vi "Dispenser Low Level.vi"(8 "error in (no error)":errorcluster, 9 "Bottom Pin":tag, 10 "Top Pin":tag="B/PWM0", 11 "Function":T1) -> (0 "error out":errorcluster)   [LabVIEW 2014]
uses:
  Controls/Dispenser Functions.ctl
  <vilib>/myRIO/Common/Instrument Driver Framework/myRIO v1.0/PWM/vis/myRIO v1.1 Open PWM.vi
  <vilib>/myRIO/Common/Instrument Driver Framework/Utilities/vis/Validate Channels.vi
  <vilib>/myRIO/Common/Instrument Driver Framework/myRIO v1.0/PWM/vis/myRIO v1.0 Reserve PWM.vi
  <vilib>/myRIO/Common/Instrument Driver Framework/myRIO v1.0/PWM/vis/myRIO v1.0 Build MUX Configuration PWM.vi
  <vilib>/myRIO/Common/Instrument Driver Framework/myRIO v1.0/Resource Manager/vis/myRIO v1.0 Reserve Channel List.vi
  <vilib>/myRIO/Common/Instrument Driver Framework/myRIO v1.0/Resource Manager/vis/myRIO v1.0 Create Configuration List.vi
  <vilib>/myRIO/Common/Instrument Driver Framework/myRIO v1.0/Resource Manager/vis/myRIO v1.0 Reserve Channel.vi
  <vilib>/myRIO/Common/Instrument Driver Framework/myRIO v1.0/Resource Manager/vis/myRIO v1.0 Unreserve Channel.vi
  <vilib>/myRIO/Common/Instrument Driver Framework/myRIO v1.0/Resource Manager/vis/myRIO v1.0 Build Mutex Name.vi
  <vilib>/Utility/VariantDataType/GetNumericInfo.vi
  <vilib>/Utility/error.llb/Error Cluster From Error Code.vi
  <vilib>/myRIO/Common/Instrument Driver Framework/myRIO v1.0/myRIO v1.1 Open.vi
  <vilib>/myRIO/Common/Instrument Driver Framework/Utilities/vis/IO Manager.vi
  <vilib>/myRIO/Common/Instrument Driver Framework/Utilities/vis/Configuration Manager.vi
  <vilib>/myRIO/Common/Instrument Driver Framework/myRIO v1.0/Resource Manager/vis/myRIO v1.0 Configure IO.vi
  <vilib>/myRIO/Common/Instrument Driver Framework/myRIO v1.0/myRIO v1.0 Close.vi
  <vilib>/myRIO/Common/Instrument Driver Framework/myRIO v1.0/PWM/vis/myRIO v1.0 Write PWM.vi
  <vilib>/myRIO/Instrument Drivers/Onboard IO/PWM/PWM.lvlib
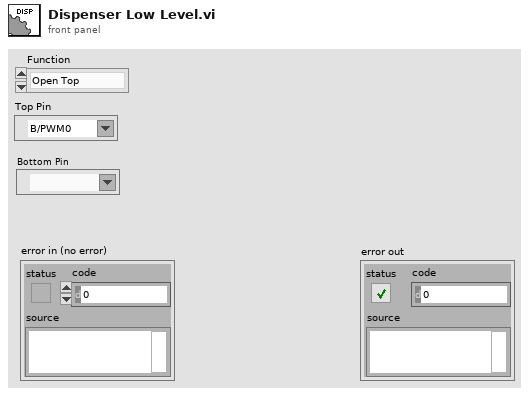
[diagram p1: front panel]
types:
  T1 = typedef "Dispenser Functions.ctl" = enum16{"Open Top", "Close Top", "Close Bottom", "Open Bottom"}
  T2 = typedef "PWM.lvlib/PWM Reference.ctl" = cluster{"myRIO Reference":T3, "PWM Channels Enum":T7, "PWM Configuration":T8}
  T3 = typedef "myRIO Generic Hardware Reference.ctl" = cluster{"myRIO Model":T4, "myRIO Hardware Reference":T5}
  T4 = typedef "Hardware Version Enum.ctl" = enum16{"Unknown", "myRIO-1900", "myRIO-1950"}
  T5 = typedef "myRIO v1.0 Reference.ctl" = cluster{"Generic FPGA Reference":T6, "Allow multiple opens":bool}
  T6 = typedef "Generic FPGA Reference.ctl" = refnum<k20>
  T7 = typedef "PWM Channels Enum.ctl" = enum16{"Not Connected", "C/PWM0", "C/PWM1", "A/PWM0", "A/PWM1", "A/PWM2", "B/PWM0", "B/PWM1", "B/PWM2"}
  T8 = typedef "PWM.lvlib/PWM Configuration.ctl" = cluster{"Frequency":dbl, "Duty Cycle":dbl}
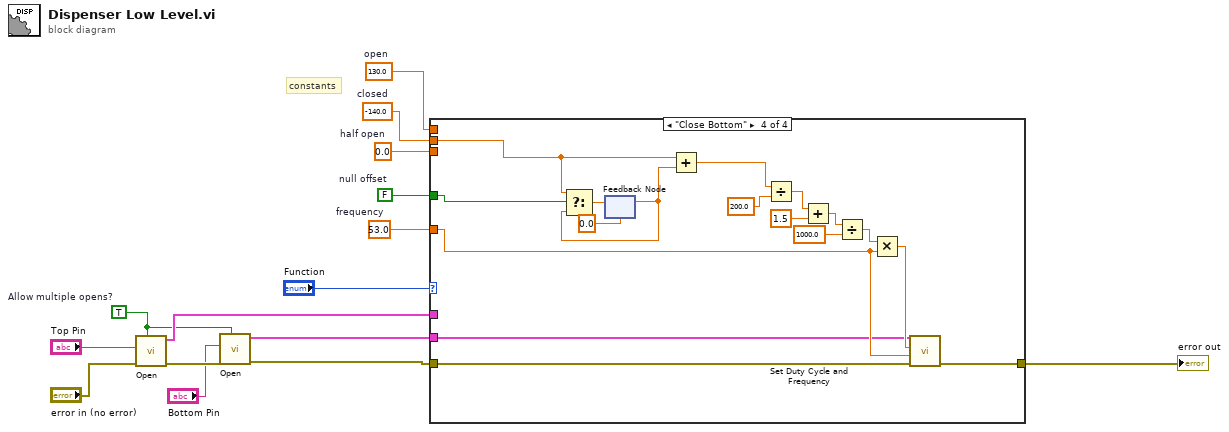
[diagram p0: block diagram]
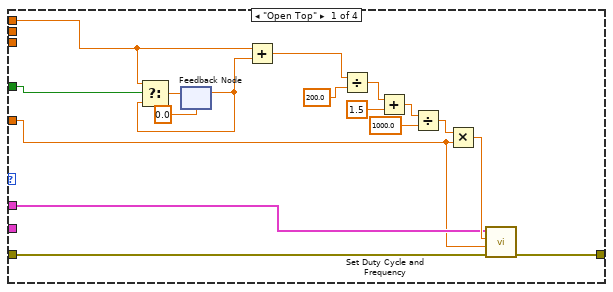
[diagram p2: hidden frame]
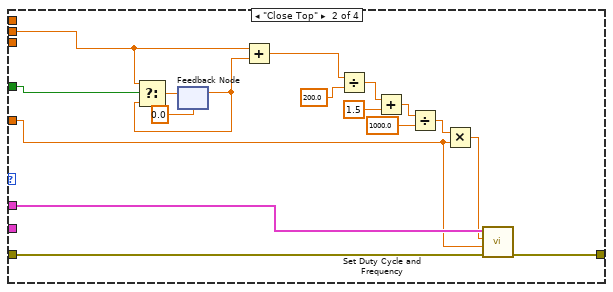
[diagram p3: hidden frame]
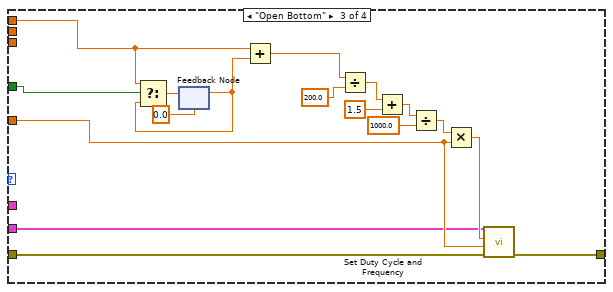
[diagram p4: hidden frame]
diagram:
  w2 = TRUE  # Allow multiple opens?
  w5 = FALSE  # null offset
  w6 = 53.0  # frequency
  w7 = 0.0  # half open
  w9 = -140.0  # closed
  w8 = 130.0  # open
  # "constants"
  n1 = call <vilib>:"Open.vi"("Allow multiple opens?"=w2, "error in (no error)"="error in (no error)", "Channel Name"="Top Pin") -> ("error out"=w12:errorcluster, "PWM Ref Out"=w3:T2)  [unwired: 7 in]
  n2 = call <vilib>:"Open.vi"("Allow multiple opens?"=w2, "error in (no error)"=w12, "Channel Name"="Bottom Pin") -> ("error out"=w11:errorcluster, "PWM Ref Out"=w4:T2)  [unwired: 7 in]
  n3 = case shown="\"Close Bottom\"" "Function" {
    tunnel: w3 -> [w19 w44 _ _]
    tunnel: w11 -> [w20 w43 w54 w72]
    tunnel: [w21 w36 w55 w71] -> w1
    tunnel: w4 -> [_ _ w50 w67]
    tunnel: w9 -> [_ w35 _ w68]
    tunnel: w8 -> [w18 _ w53 _]
    tunnel: w7 -> [_ _ _ _]
    tunnel: w6 -> [w16 w34 w51 w70]
    tunnel: w5 -> [w17 w33 w52 w69]
    frame "Open Top" {
      n4 = feedback #1(0.0 ("position [%FS]")) -> (w29:dbl)
      n5 = Select(t=w18, s=w17, f=w29) -> (s? t:f=w27:dbl)
      n6 = feedback-in #1(w27) -> ()
      n7 = Add(x=w18, y=w29) -> (x+y=w28:dbl)
      n8 = Divide(x=w28, y=200.0) -> (x/y=w23:dbl)
      n9 = Add(x=w23, y=1.5) -> (x+y=w25:dbl)
      n10 = Divide(x=w25, y=1000.0) -> (x/y=w30:dbl)
      n11 = Multiply(x=w30, y=w16) -> (x*y=w31:dbl)
      n12 = call <vilib>:"Set Duty Cycle and Frequency.vi"("error in (no error)"=w20, "Frequency [Hz]"=w16, "Duty Cycle"=w31, "PWM Ref In"=w19) -> ("error out"=w21:errorcluster)  [unwired: 5 in, 1 out]
    }
    frame "Close Top" {
      n13 = feedback #2(0.0 ("position [%FS]")) -> (w40:dbl)
      n14 = Select(t=w35, s=w33, f=w40) -> (s? t:f=w42:dbl)
      n15 = feedback-in #2(w42) -> ()
      n16 = Add(x=w35, y=w40) -> (x+y=w41:dbl)
      n17 = Divide(x=w41, y=200.0) -> (x/y=w48:dbl)
      n18 = Add(x=w48, y=1.5) -> (x+y=w46:dbl)
      n19 = Divide(x=w46, y=1000.0) -> (x/y=w39:dbl)
      n20 = Multiply(x=w39, y=w34) -> (x*y=w38:dbl)
      n21 = call <vilib>:"Set Duty Cycle and Frequency.vi"("error in (no error)"=w43, "Frequency [Hz]"=w34, "Duty Cycle"=w38, "PWM Ref In"=w44) -> ("error out"=w36:errorcluster)  [unwired: 5 in, 1 out]
    }
    frame "Open Bottom" {
      n22 = feedback #3(0.0 ("position [%FS]")) -> (w63:dbl)
      n23 = Select(t=w53, s=w52, f=w63) -> (s? t:f=w61:dbl)
      n24 = feedback-in #3(w61) -> ()
      n25 = Add(x=w53, y=w63) -> (x+y=w62:dbl)
      n26 = Divide(x=w62, y=200.0) -> (x/y=w57:dbl)
      n27 = Add(x=w57, y=1.5) -> (x+y=w59:dbl)
      n28 = Divide(x=w59, y=1000.0) -> (x/y=w64:dbl)
      n29 = Multiply(x=w64, y=w51) -> (x*y=w65:dbl)
      n30 = call <vilib>:"Set Duty Cycle and Frequency.vi"("error in (no error)"=w54, "Frequency [Hz]"=w51, "Duty Cycle"=w65, "PWM Ref In"=w50) -> ("error out"=w55:errorcluster)  [unwired: 5 in, 1 out]
    }
    frame "Close Bottom" {
      n31 = feedback #4(0.0 ("position [%FS]")) -> (w80:dbl)
      n32 = Select(t=w68, s=w69, f=w80) -> (s? t:f=w78:dbl)
      n33 = feedback-in #4(w78) -> ()
      n34 = Add(x=w68, y=w80) -> (x+y=w79:dbl)
      n35 = Divide(x=w79, y=200.0) -> (x/y=w74:dbl)
      n36 = Add(x=w74, y=1.5) -> (x+y=w76:dbl)
      n37 = Divide(x=w76, y=1000.0) -> (x/y=w81:dbl)
      n38 = Multiply(x=w81, y=w70) -> (x*y=w82:dbl)
      n39 = call <vilib>:"Set Duty Cycle and Frequency.vi"("error in (no error)"=w72, "Frequency [Hz]"=w70, "Duty Cycle"=w82, "PWM Ref In"=w67) -> ("error out"=w71:errorcluster)  [unwired: 5 in, 1 out]
    }
  }
  "error out" <- w1
